vi "drive control (IO).vi"(1 "velocity":i16, 2 "drive vector":i8) -> ()   [LabVIEW 2009]
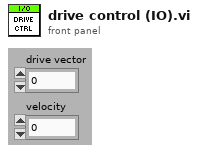
[diagram p1: front panel]
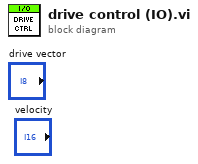
[diagram p0: block diagram]
diagram:
